vi "delete_start_scan.vi"(10 "error out":errorcluster, 11 "base path":path) -> (3 "error out 2":errorcluster)   [LabVIEW 2018]
panel:
  out "file or folder exists?":bool
  out "appended path":path
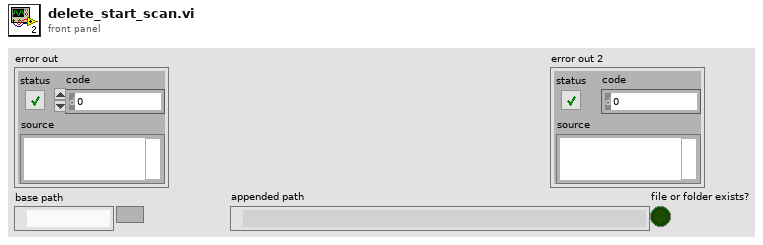
[diagram p1: front panel]
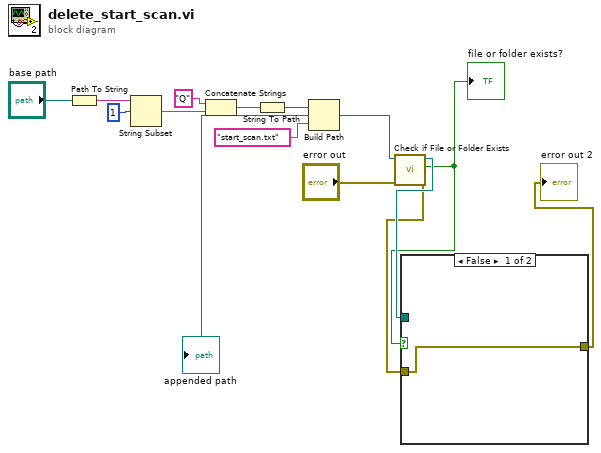
[diagram p0: block diagram]
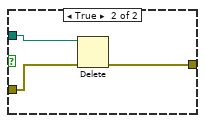
[diagram p2: hidden frame]
diagram:
  n1 = Path To String(path="base path") -> (string=w10:string)
  n2 = String Subset(string=w10, offset (0)=1) -> (substring=w7:string)  [unwired: 1 in]
  n3 = Concatenate Strings("Q" ("string"), w7) -> (w6:string)
  n4 = String To Path(string=w6) -> (path=w5:path)
  n5 = Build Path(base path=w5, name or relative path="start_scan.txt") -> (appended path=w14:path)
  "appended path" <- w14
  n6 = call <vilib>:"Check if File or Folder Exists.vi"("error in (no error)"="error out", "path"=w14) -> ("error out"=w2:errorcluster, "file or folder exists?"=w3:bool, "dup path"=w4:path)  [unwired: 7 in]
  "file or folder exists?" <- w3
  n7 = case shown="False" w3 {
    tunnel: w4 -> [_ w18]
    tunnel: w2 -> [w15 w17]
    tunnel: [w15 w16] -> w1
    frame False {
    }
    frame True {
      n8 = Delete(path (use dialog)=w18, error in=w17) -> (error out=w16:errorcluster)  [unwired: 3 in, 2 out]
    }
  }
  "error out 2" <- w1
